vi "Test Simple Server.vi"() -> ()   [LabVIEW 2020]
uses:
  Test Index/Test Index.lvclass
  C:/Program Files (x86)/National Instruments/LabVIEW 2020/vi.lib/IlluminatedG/IG HTTP Server/HTTP Server/Handler/Handler.lvclass
  <vilib>/IlluminatedG/IG HTTP Server/HTTP Server/Server/Add Connection Handler.vi
  <vilib>/IlluminatedG/IG HTTP Server/HTTP Server/Server/Add Request Handler.vi
  <vilib>/IlluminatedG/IG HTTP Server/HTTP Server/Server/Add Route Handler.vi
  <vilib>/IlluminatedG/IG HTTP Server/HTTP Server/Server/Add Controller Handler.vi
  <vilib>/IlluminatedG/IG HTTP Server/HTTP Server/Server/Add Controller.vi
  <vilib>/IlluminatedG/IG HTTP Server/HTTP Server/Server/Add Response Handler.vi
  <vilib>/IlluminatedG/IG HTTP Server/HTTP Server/Server/Add Complete Handler.vi
  <vilib>/IlluminatedG/IG HTTP Server/HTTP Server/Server/Add Exception Handler.vi
  <vilib>/IlluminatedG/IG HTTP Server/HTTP Server/Connection Handler/Connection Handler.lvclass
  <vilib>/IlluminatedG/IG HTTP Server/HTTP Server/Request Handler/Request Handler.lvclass
  <vilib>/IlluminatedG/IG HTTP Server/HTTP Server/Route Handler/Route Handler.lvclass
  <vilib>/IlluminatedG/IG HTTP Server/HTTP Server/Controller Handler/Controller Handler.lvclass
  <vilib>/IlluminatedG/IG HTTP Server/HTTP Server/Controller/Controller.lvclass
  <vilib>/IlluminatedG/IG HTTP Server/HTTP Server/Response Handler/Response Handler.lvclass
  <vilib>/IlluminatedG/IG HTTP Server/HTTP Server/Complete Handler/Complete Handler.lvclass
  <vilib>/IlluminatedG/IG HTTP Server/HTTP Server/Exception Handler/Exception Handler.lvclass
  <vilib>/IlluminatedG/IG HTTP Server/HTTP Server/Server/Server.lvclass
  <vilib>/IlluminatedG/IG HTTP Server/HTTP Server/Handler/Handler.lvclass
panel:
  out "error out":errorcluster
  in  "Port":u16=36987
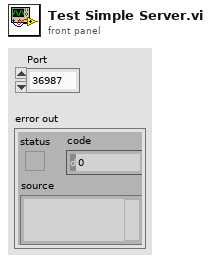
[diagram p1: front panel]
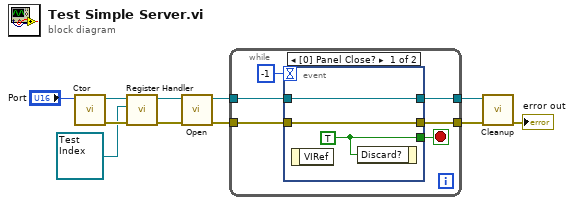
[diagram p0: block diagram]
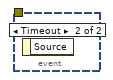
[diagram p2: hidden frame]
diagram:
  n1 = call <vilib>:"Ctor.vi"("HTTP Port (80)"="Port") -> ("error out"=w2:errorcluster, "Server out"=w5:refnum<class "Server.lvclass">)  [unwired: 9 in]
  n2 = call <vilib>:"Register Handler.vi"("error in (no error)"=w2, "Handler"=refnum<class "Test Index.lvclass"> refnum ("Test Index.lvclass"), "Server in"=w5) -> ("error out"=w3:errorcluster, "Server out"=w4:refnum<class "Server.lvclass">)  [unwired: 7 in]
  n3 = call <vilib>:"Open.vi"("error in (no error)"=w3, "Server in"=w4) -> ("error out"=w9:errorcluster, "Server out"=w10:refnum<class "Server.lvclass">)  [unwired: 8 in]
  n4 = while {
    tunnel: w10 -> [w15]
    tunnel: w9 -> [w16]
    tunnel: [w14] -> w8
    tunnel: [w13] -> w7
    stop <- w17 stop-if-true
    n5 = event shown="[0] Panel Close?" {
      selector: _ -> [_ _]
      dyn-events: _ -> [_ _]
      timeout: -1 -> [_ _]
      tunnel: [w20 _] -> w17
      tunnel: w16 -> [w18 _]
      tunnel: w15 -> [w19 _]
      tunnel: [w19 _] -> w14
      tunnel: [w18 _] -> w13
      event Panel Close? {
        w20 = TRUE ("Discard?")
        n6 = event-data() -> ()  [unwired: 1 in, 1 out]
        n7 = event-data("Discard?"=w20) -> ()  [unwired: 1 in, 1 out]
      }
      event Timeout {
        n8 = event-data() -> ()  [unwired: 1 in, 1 out]
      }
    }
  }
  n9 = call <vilib>:"Cleanup.vi"("error in (no error)"=w7, "Server in"=w8) -> ("error out"=→"error out":errorcluster)  [unwired: 9 in]
